vi "Page Hiearchy to Title.vi"(11 "Page Hierarchy":string[](array[string])) -> (3 "Page Title":string)   [LabVIEW 2023, in "VIDoc Printer - Confluence.lvlib" / "VIDoc Printer - Confluence.lvclass"]
uses:
  VIDoc Printer - Confluence.lvclass
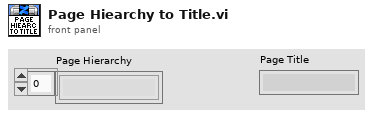
[diagram p1: front panel]
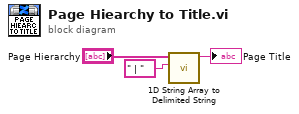
[diagram p0: block diagram]
diagram:
  n1 = call <vilib>:"1D String Array to Delimited String.vi"("delimiter"=" | ", "string array"="Page Hierarchy") -> ("delimited string"=→"Page Title":string)  [unwired: 9 in]
